vi "jettl Msg Template.vi"() -> (2 "Msg Strategy":refnum<class "Msg Strategy.lvclass">)   [LabVIEW 2021, in "jettl Msg Template.lvlib"]
uses:
  jettl Msg Template.lvlib
  <vilib>/jettl/jettl/jettl/Msg Strategy/Msg Strategy.lvclass
  Template Msg Strategy/Template Msg Strategy.lvclass
  C:/Program Files/National Instruments/LabVIEW 2021/vi.lib/jettl/jettl/jettl/Msg Strategy/Msg Strategy.lvclass
  C:/Program Files/National Instruments/LabVIEW 2021/project/jettl/_Template/Templates/jettl Msg Template/Template Msg Strategy/Template Msg Strategy.lvclass
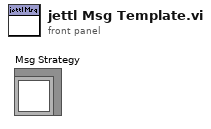
[diagram p1: front panel]
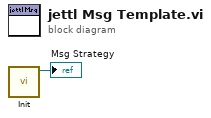
[diagram p0: block diagram]
diagram:
  n1 = call "Init.vi"() -> ("Template Msg Strategy out"=→"Msg Strategy":refnum<class "Template Msg Strategy.lvclass">)  [unwired: 11 in]
